vi "IHM_SetStringValue.vi"(4 "error in (no error)":errorcluster caption="entrée d'erreur (pas d'erreur)", 6 "StringValue":string, 7 "Ref_IN":T1) -> (0 "Error out":errorcluster, 3 "Ref_OUT":T1)   [LabVIEW 2013]
panel:
  out "ClassName":string
  out "Name":string
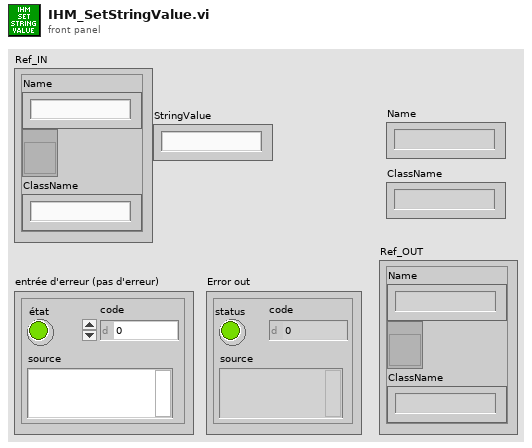
[diagram p1: front panel]
types:
  T1 = cluster{"Name":string, refnum<vi>, "ClassName":string}
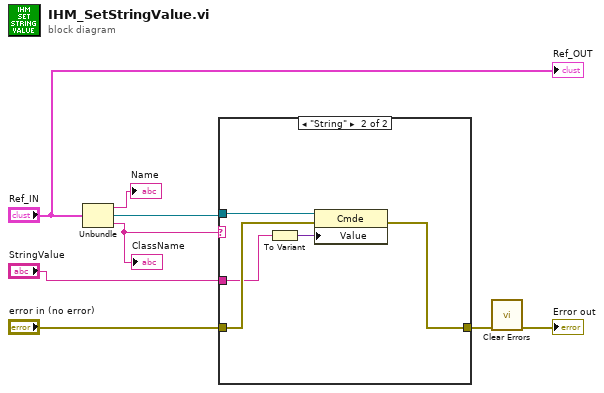
[diagram p0: block diagram]
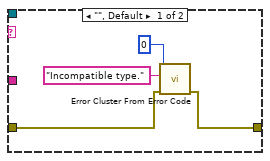
[diagram p2: hidden frame]
diagram:
  n1 = Unbundle("Ref_IN") -> ("Name"=→"Name":string, w7:refnum<vi>, "ClassName"=w8:string)
  "ClassName" <- w8
  n2 = case shown="\"String\"" w8 {
    tunnel: w7 -> [_ w17]
    tunnel: "error in (no error)" -> [w12 w15]
    tunnel: [w11 w14] -> w3
    tunnel: "StringValue" -> [_ w13]
    frame "", Default {
      n3 = call <vilib>:"Error Cluster From Error Code.vi"("error in (no error)"=w12, "error message (\"\")"="Incompatible type." ("error message (\"\")"), "error code (0)"=0) -> ("error out"=w11:errorcluster)  [unwired: 6 in]
    }
    frame "String" {
      n4 = To Variant(anything=w13) -> (Variant=w16:variant)
      n5 = property class="Cmde"(reference=w17, error in=w15, "Value"=w16) -> (error out=w14:errorcluster)  [unwired: 1 out]
    }
  }
  n6 = call <vilib>:"Clear Errors.vi"("error in (no error)"=w3) -> ("error out"=→"Error out":errorcluster)  [unwired: 6 in]
  "Ref_OUT" <- "Ref_IN"
